vi "W7-X-Bolo-TMDS-LOCAL.vi"(0 "Kappa 2":dbl[](array[numeric]), 1 "ArrayOutput 4":dbl[](array[numeric]), 2 "ArrayOutput 3":dbl[](array[numeric]), 3 "Array":sgl[][](array[numeric]), 5 "RawArray":sgl[][](array[numeric]), 7 "Numeric":sgl, 9 "ArrayOutput":dbl[](array[numeric]), 12 "Kappa":dbl[](array[numeric]), 13 "ArrayOutput 2":dbl[](array[numeric]), 14 "SampleTime":sgl) -> (15 "error out":errorcluster)   [LabVIEW 2014]
uses:
  <vilib>/Utility/file.llb/Write To Spreadsheet File (DBL).vi
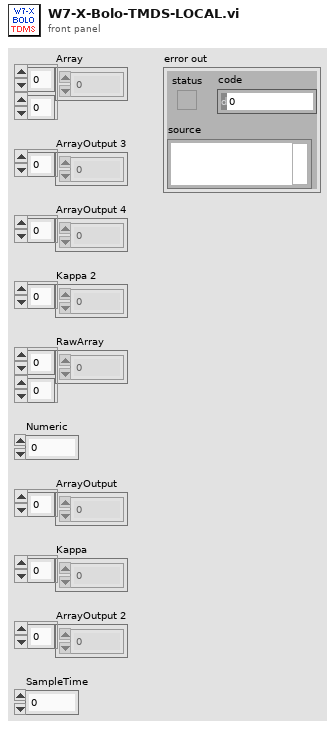
[diagram p1: front panel]
types:
  T1 = enum16{"open", "open or create", "create or replace", "create", "open (read-only)"}
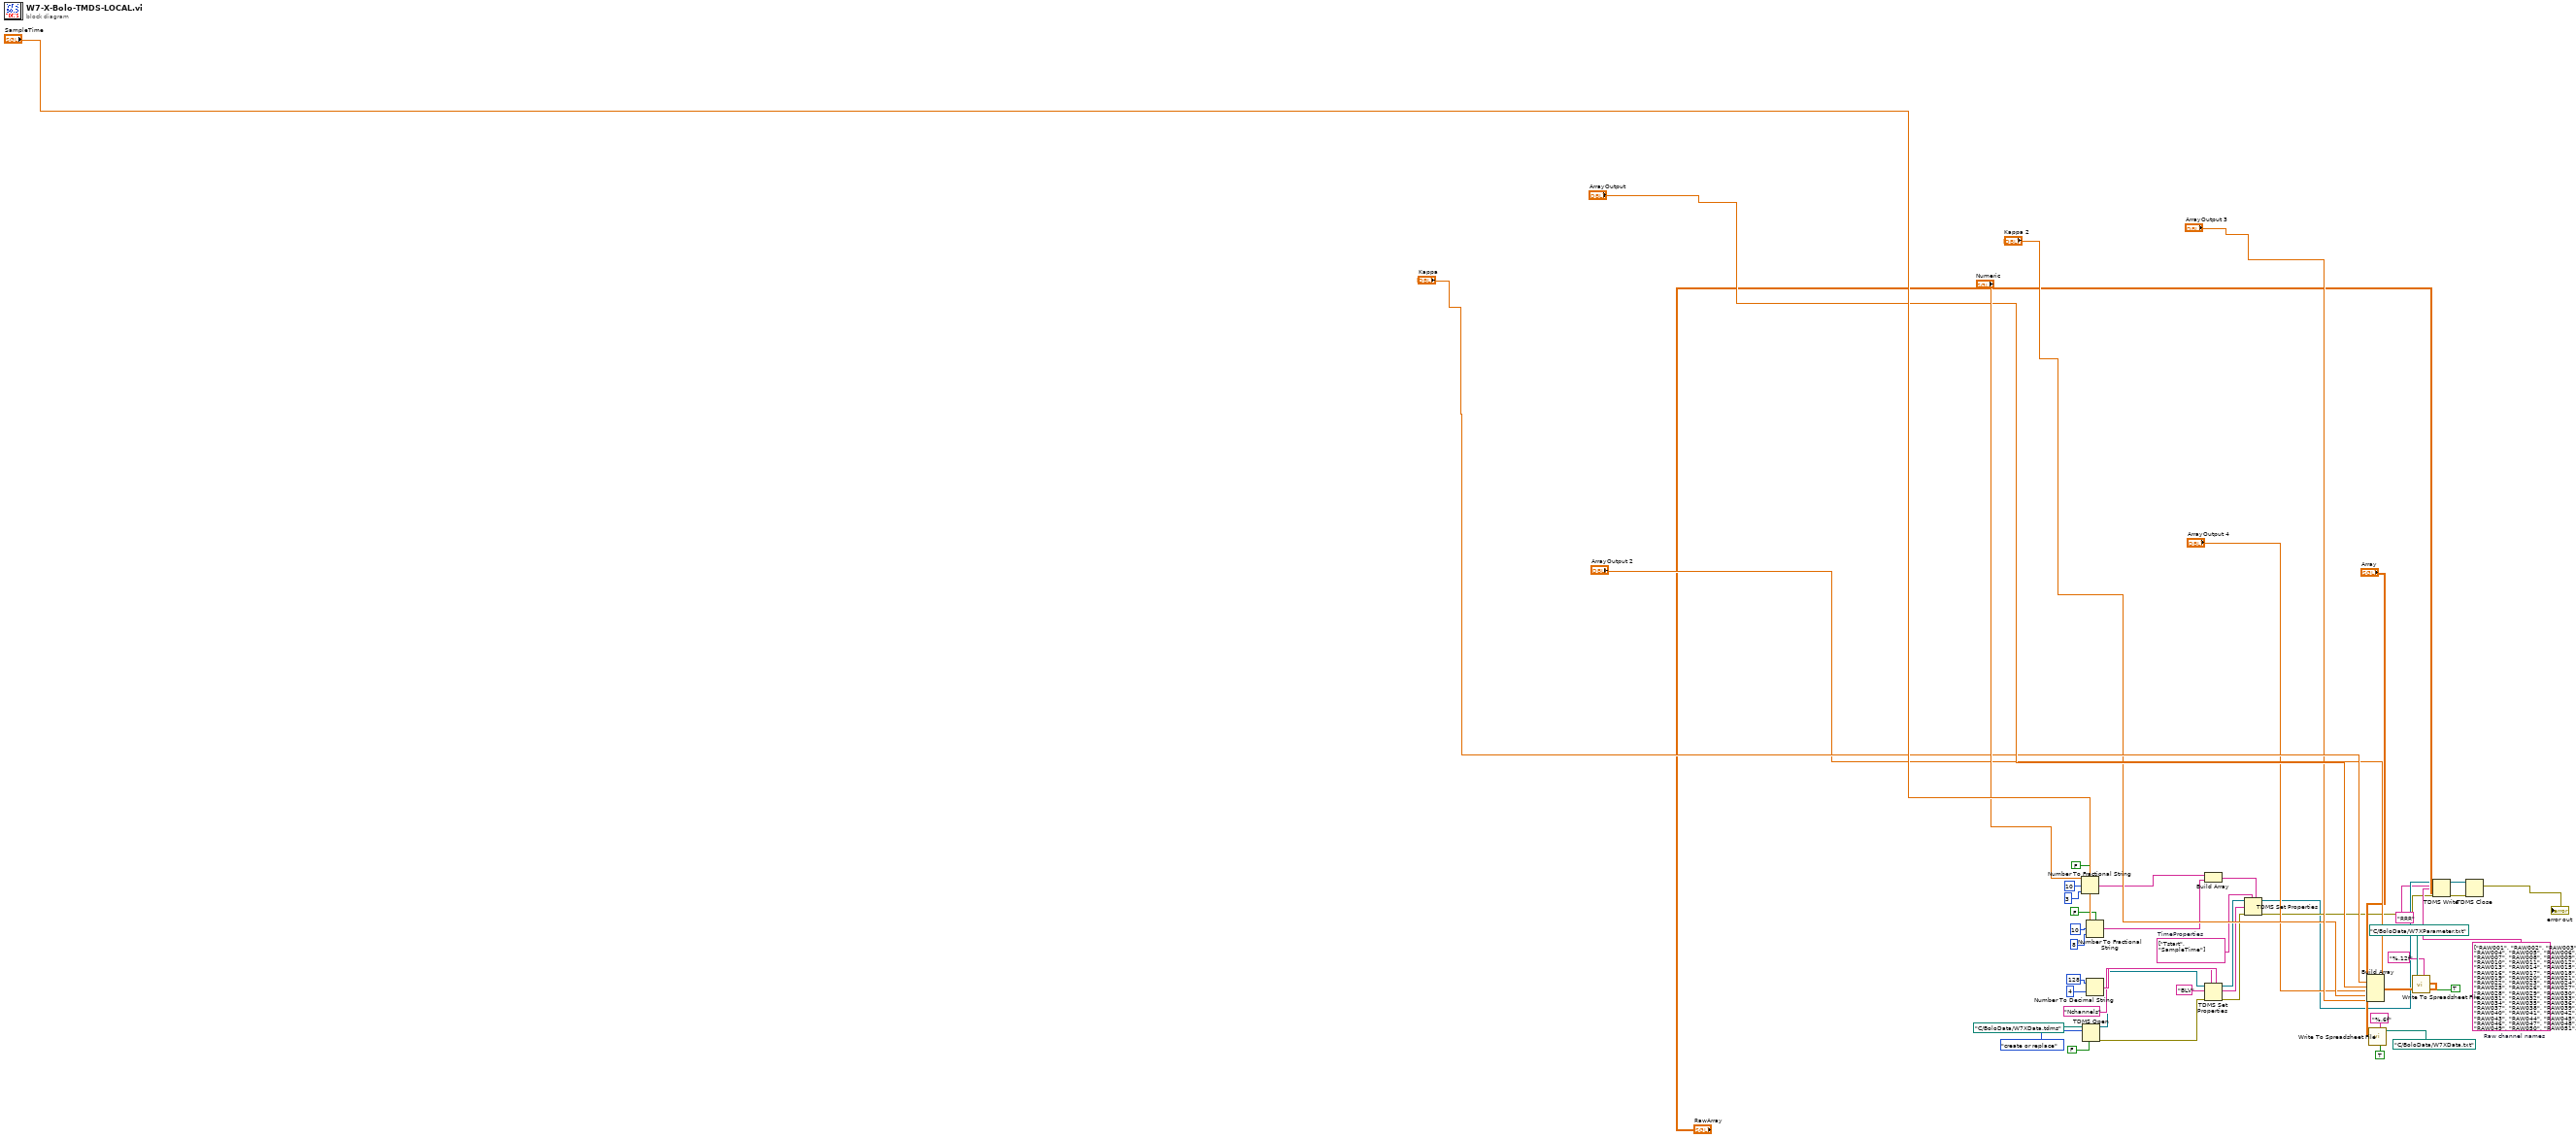
[diagram p0: block diagram]
diagram:
  w26 = string[] ["RAW001", "RAW002", "RAW003", "RAW004", "RAW005", "RAW006", "RAW007", "RAW008", "RAW009", "RAW010", "RAW011", "RAW012", "RAW013", "RAW014", "RAW015", "RAW016", "RAW017", "RAW018", "RAW019", "RAW020", "RAW021", "RAW022", "RAW023", "RAW024", "RAW025", "RAW026", "RAW027", "RAW028", "RAW029", "RAW030", "RAW031", "RAW032", "RAW033", "RAW034", "RAW035", "RAW036", "RAW037", "RAW038", "RAW039", "RAW040", "RAW041", "RAW042", "RAW043", "RAW044", "RAW045", "RAW046", "RAW047", "RAW048", "RAW049", "RAW050", "RAW051", "RAW052", "RAW053", "RAW054", "RAW055", "RAW056", "RAW057", "RAW058", "RAW059", "RAW060", "RAW061", "RAW062", "RAW063", "RAW064", "RAW065", "RAW066", "RAW067", "RAW068", "RAW069", "RAW070", "RAW071", "RAW072", "RAW073", "RAW074", "RAW075", "RAW076", "RAW077", "RAW078", "RAW079", "RAW080", "RAW081", "RAW082", "RAW083", "RAW084", "RAW085", "RAW086", "RAW087", "RAW088", "RAW089", "RAW090", "RAW091", "RAW092", "RAW093", "RAW094", "RAW095", "RAW096", "RAW097", "RAW098", "RAW099", "RAW100", "RAW101", "RAW102", "RAW103", "RAW104", "RAW105", "RAW106", "RAW107", "RAW108", "RAW109", "RAW110", "RAW111", "RAW112", "RAW113", "RAW114", "RAW115", "RAW116", "RAW117", "RAW118", "RAW119", "RAW120", "RAW121", "RAW122", "RAW123", "RAW124", "RAW125", "RAW126", "RAW127", "RAW128"]  # Raw channel names
  w8 = string[] ["Tstart", "SampleTime"]  # TimeProperties
  n1 = Number To Fractional String(use system decimal point (T)=FALSE, number="Numeric", width (-)=i16 10, precision (6)=i16 3) -> (F-format string=w9:string)
  n2 = TDMS Open(6:FALSE ("disable buffering? (T)"), 10:T1."create or replace" ("operation (0:open)"), 11:path "C:/BoloData/W7XData.tdms" ("file path")) -> (0:w11:errorcluster, 3:w17:refnum<k34>)  [unwired: 4 in]
  n3 = Number To Fractional String(use system decimal point (T)=FALSE, number="SampleTime", width (-)=i16 10, precision (6)=i16 8) -> (F-format string=w7:string)
  n4 = Number To Decimal String(number=128 ("Channels"), width (-)=i16 4) -> (decimal integer string=w21:string)
  n5 = TDMS Set Properties(5:w21, 7:"Nchannels" ("DiagnosticProperties"), 8:w11, 10:"BLV" ("group name"), 11:w17) -> (0:w10:errorcluster, 2:w13:string, 3:w18:refnum<k34>)  [unwired: 2 out]
  n6 = Build Array(w9, w7) -> (w6:string[])
  n7 = TDMS Set Properties(5:w6, 7:w8, 8:w10, 10:w13, 11:w18) -> (0:w25:errorcluster, 3:w24:refnum<k34>)  [unwired: 3 out]
  n8 = Build Array("ArrayOutput 2", "Kappa", "ArrayOutput", "ArrayOutput 4", "Kappa 2", "ArrayOutput 3") -> (w42:dbl[][])
  n9 = call-poly <vilib>:"Write To Spreadsheet File.vi"("transpose? (no:F)"=TRUE, "format (%.3f)"="%.6f", "2D data"="Array", "file path (dialog if empty)"=path "C:/BoloData/W7XData.txt" ("file path")) -> ()  [unwired: 4 in, 1 out]
  n10 = call-poly <vilib>:"Write To Spreadsheet File.vi"("transpose? (no:F)"=TRUE, "format (%.3f)"="%.12f", "2D data"=w42, "file path (dialog if empty)"=path "C:/BoloData/W7XParameter.txt" ("file path")) -> ()  [unwired: 4 in, 1 out]
  n11 = TDMS Write(0:w24, 5:"RRR" ("group name in (Untitled)"), 7:w26, 9:"RawArray", 11:w25) -> (4:w27:refnum<k34>, 15:w28:errorcluster)  [unwired: 1 in, 2 out]
  n12 = TDMS Close(8:w28, 11:w27) -> (0:→"error out":errorcluster)  [unwired: 1 out]
